vi "ParseSegments.vi"(11 "path":string) -> (2 "invalid":bool, 3 "Segments":string[](array[string]))   [LabVIEW 2013, in "openURI.lvlib"]
uses:
  openURI.lvlib
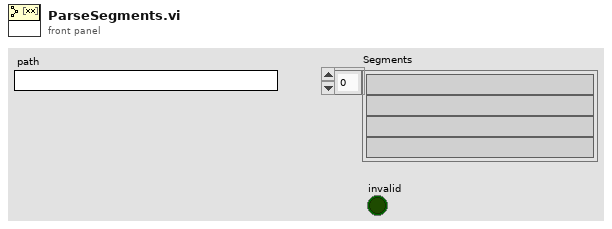
[diagram p1: front panel]
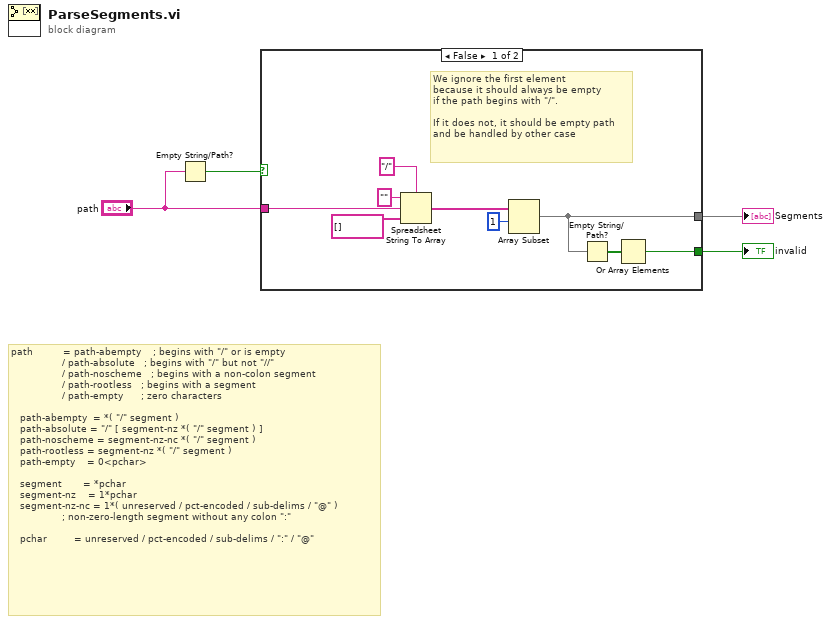
[diagram p0: block diagram]
diagram:
  # "path          = path-abempty    ; begins with \"/\" or is empty\n                 / path-absolute   ; begins with \"/\" but not \"//\"\n                 / path-noscheme   ; begins with a non-colon segment\n                 / path-rootless   ; begins with a segment\n                 / path-empty      ; zero characters\n\n   path-abempty  = *( \"/\" segment )\n   path-absolute = \"/\" [ segment-nz *( \"/\" segment ) ]\n   path-noscheme = segment-nz-nc *( \"/\" segment )\n   path-rootless = segment-nz *( \"/\" segment )\n   path-empty    = 0<pchar>\n\n   segment       = *pchar\n   segment-nz    = 1*pchar\n   segment-nz-nc = 1*( unreserved / pct-encoded / sub-delims / \"@\" )\n                 ; non-zero-length segment without any colon \":\"\n\n   pchar         = unreserved / pct-encoded / sub-delims / \":\" / \"@\""
  n1 = Empty String/Path?(string/path="path") -> (empty?=w2:bool)
  n2 = case shown="False" w2 {
    tunnel: [w7 _] -> w4
    tunnel: "path" -> [w8 _]
    tunnel: [w5 _] -> w1
    frame False {
      # "We ignore the first element\nbecause it should always be empty\nif the path begins with \"/\".\n\nIf it does not, it should be empty path\nand be handled by other case"
      n3 = Spreadsheet String To Array(delimiter (Tab)="/", format string="", spreadsheet string=w8, array type (2D Dbl)=string[] [] ("Segments")) -> (array=w9:string[])
      n4 = Array Subset(array=w9, index=1) -> (w7:string[])  [unwired: 1 in]
      n5 = Empty String/Path?(string/path=w7) -> (empty?=w6:bool[])
      n6 = Or Array Elements(Boolean array=w6) -> (logical OR=w5:bool)
    }
    frame True {
    }
  }
  "Segments" <- w4
  "invalid" <- w1
